vi "Read ReleaseDate.vi"(8 "error in (no error)":errorcluster, 11 "Package Version in":refnum<class "Package Version.lvclass">) -> (0 "error out":errorcluster, 2 "ReleaseDate":timestamp, 3 "Package Version out":refnum<class "Package Version.lvclass">)   [LabVIEW 2020, in "Packages.lvlib" / "Package Version.lvclass"]
uses:
  Package Version.lvclass
  Package Version.lvclass/Package Version.ctl
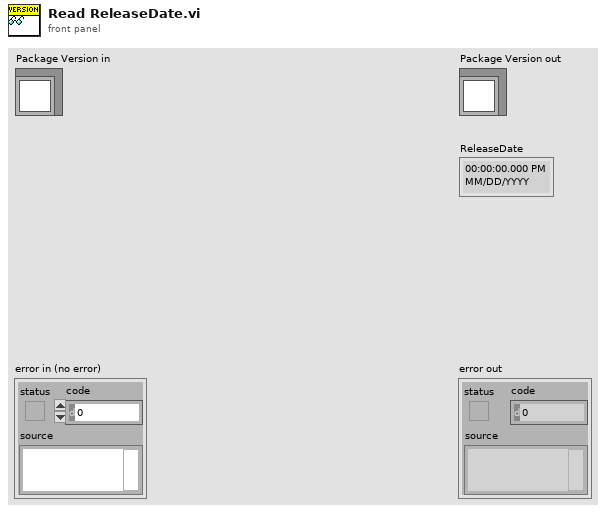
[diagram p1: front panel]
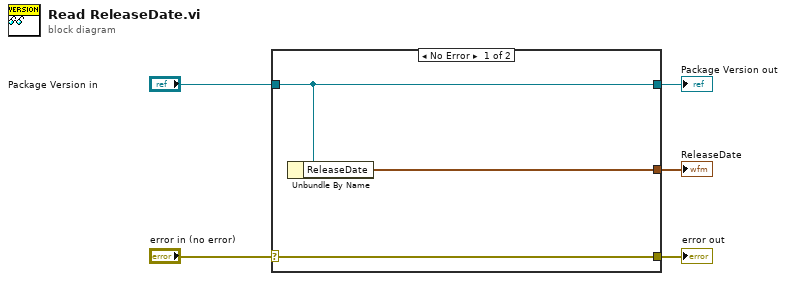
[diagram p0: block diagram]
diagram:
  n1 = case shown="No Error" "error in (no error)" {
    selector: "error in (no error)" -> [w8 w9]
    tunnel: [w8 w9] -> w4
    tunnel: [w7 w10] -> w2
    tunnel: "Package Version in" -> [w7 w10]
    tunnel: [w6 _] -> w1
    frame No Error {
      n2 = Unbundle By Name(w7) -> ("ReleaseDate"=w6:timestamp)
    }
    frame Error {
    }
  }
  "error out" <- w4
  "Package Version out" <- w2
  "ReleaseDate" <- w1
